vi "Bind Boolean Text.vi"(5 "Data Type":variant, 6 "Format String":string, 7 "Bind by Label (F=Bind by Caption)":bool, 8 "error in (no error)":errorcluster, 9 "Datum Name (Use Control Text)":string, 10 "Bool Refnum":refnum<vi>, 11 "IObserver in":refnum<class "IObserver.lvclass">) -> (0 "error out":errorcluster, 3 "IObserver out":refnum<class "IObserver.lvclass">)   [LabVIEW 2015, in "IObserver.lvlib" / "IObserver.lvclass"]
doc: "<License>\nCopyright © 2017 Composed Systems, LLC | All rights reserved\nwww.composed.io\n\nAuthor: Ethan Stern <ethan.stern@composed.io>\n\nThis software is provided \"AS IS\" WITHOUT WARRANTIES, either express or implied, AND IS FOR EDUCATIONAL PURPOSES ONLY.\n</License>"
uses:
  IObserver.lvclass
  <vilib>/ActorFramework/Actor/Actor.lvclass/Actor.ctl
  <vilib>/ActorFramework/Message Enqueuer/Message Enqueuer.lvclass/Message Enqueuer.ctl
  SubscriptionPolicy/ValueChangeSubscription/ValueChangeSubscription.lvclass/ValueChangeSubscription.ctl
  IObserver Messages/Subscribe Msg/Subscribe Msg.lvclass/Subscribe Msg.ctl
  <vilib>/ActorFramework/Message Enqueuer/Init from Existing Queue.vi
  <vilib>/ActorFramework/Message Enqueuer/Enqueue.vi
  <vilib>/ActorFramework/Message Priority Queue/Priority Enqueue.vi
  <vilib>/ActorFramework/Message Enqueuer/Message Enqueuer.lvclass
  SubscriptionPolicy/ValueChangeSubscription/ValueChangeSubscription.lvclass
  IObserver Messages/Subscribe Msg/Subscribe Msg.lvclass
  IMediator/SubscriptionRequest/SubscriptionRequest.lvclass
  <vilib>/ActorFramework/Actor/Actor.lvclass
  Transport/BooleanTextBinding/BooleanTextBinding.lvclass
  IMediator/ISubscriptionPolicy/ISubscriptionPolicy.lvclass
panel:
  in  "Ignore Past Updates? (F)":bool
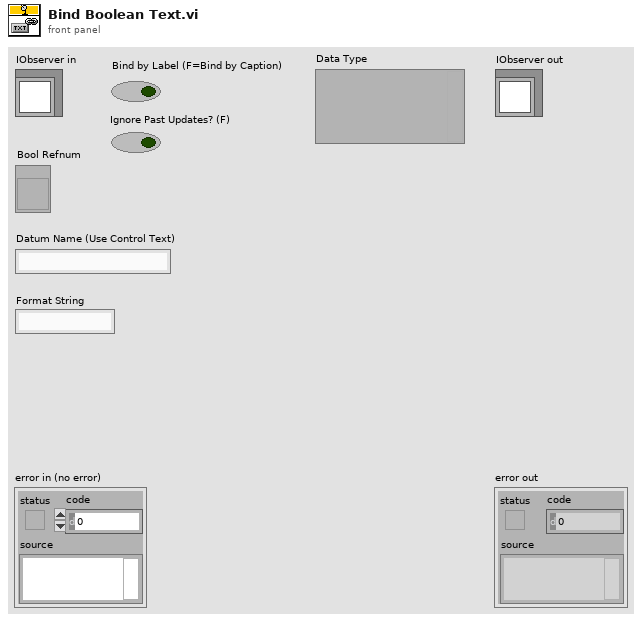
[diagram p1: front panel]
types:
  T1 = typedef "IMediator.lvlib/ISubscriptionPolicy.lvclass/ISubscriptionPolicy Reference.ctl" = refnum<data-value>
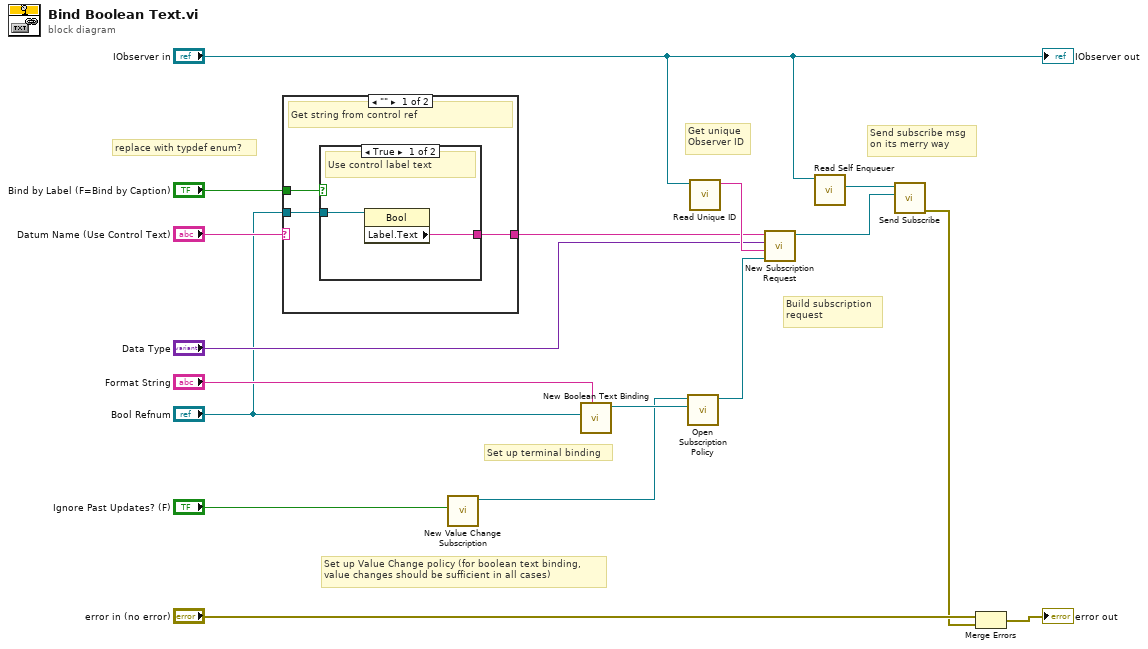
[diagram p0: block diagram]
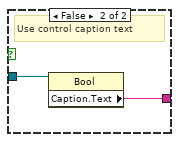
[diagram p2: hidden frame]
diagram:
  # "Set up Value Change policy (for boolean text binding,\nvalue changes should be sufficient in all cases)"
  # "replace with typdef enum?"
  # "Send subscribe msg\non its merry way"
  # "Build subscription\nrequest"
  # "Get unique\nObserver ID"
  # "Set up terminal binding"
  n1 = case shown="\"\"" "Datum Name (Use Control Text)" {
    selector: "Datum Name (Use Control Text)" -> [_ w25]
    tunnel: [w18 w25] -> w9
    tunnel: "Bind by Label (F=Bind by Caption)" -> [w20 _]
    tunnel: "Bool Refnum" -> [w19 _]
    frame "" {
      # "Get string from control ref"
      n2 = case shown="True" w20 {
        tunnel: w19 -> [w22 w24]
        tunnel: [w21 w23] -> w18
        frame True {
          # "Use control label text"
          n3 = property class="Bool"(reference=w22) -> ("Label.Text"=w21:string)  [unwired: 1 in, 2 out]
        }
        frame False {
          # "Use control caption text"
          n4 = property class="Bool"(reference=w24) -> ("Caption.Text"=w23:string)  [unwired: 1 in, 2 out]
        }
      }
    }
    frame Default {
      # "Use string wired to input terminal"
    }
  }
  n5 = call "New Value Change Subscription.vi"("Ignore Past Updates? (F)"="Ignore Past Updates? (F)") -> ("ValueChangeSubscription Out"=w1:refnum<class "ValueChangeSubscription.lvclass">)  [unwired: 10 in]
  n6 = call "New Boolean Text Binding.vi"("Format String"="Format String", "Bool Refnum"="Bool Refnum") -> ("BooleanTextBinding Out"=w4:refnum<class "BooleanTextBinding.lvclass">)  [unwired: 8 in, 1 out]
  n7 = call "Open Subscription Policy.vi"("Transport"=w4, "SubscriptionPolicy"=w1) -> ("Subscription Policy"=w5:T1)  [unwired: 8 in, 1 out]
  n8 = call "Read Unique ID.vi"("IObserver In"="IObserver in") -> ("Unique ID"=w16:string)  [unwired: 10 in]
  n9 = call "New Subscription Request.vi"("Subscription Policy"=w5, "Subscriber ID"=w16, "Type"="Data Type", "Datum Name"=w9) -> ("SubscriptionRequest"=w3:refnum<class "SubscriptionRequest.lvclass">)  [unwired: 7 in]
  n10 = call <vilib>:"Read Self Enqueuer.vi"("Actor"="IObserver in") -> ("Self Enqueuer"=w14:refnum<class "Message Enqueuer.lvclass">)  [unwired: 10 in]
  n11 = call "Send Subscribe.vi"("SubscriptionRequest"=w3, "Message Enqueuer"=w14) -> ("error out"=w12:errorcluster)  [unwired: 8 in, 1 out]
  n12 = Merge Errors("error in (no error)", w12) -> (→"error out":errorcluster)
  "IObserver out" <- "IObserver in"
